vi "Get Conditional Column Data.vi"(4 "Condition Header Value":string, 6 "Condition Header":string, 8 "error in (no error)":errorcluster, 10 "Header":string, 11 "SLL Table in":refnum<class "SLL Table.lvclass">) -> (0 "error out":errorcluster, 2 "Data[]":string[](array[string]), 3 "SLL Table out":refnum<class "SLL Table.lvclass">)   [LabVIEW 2014, in "SLL Table.lvclass"]
uses:
  SLL Table.lvclass
  SLL String/SLL String.lvlib
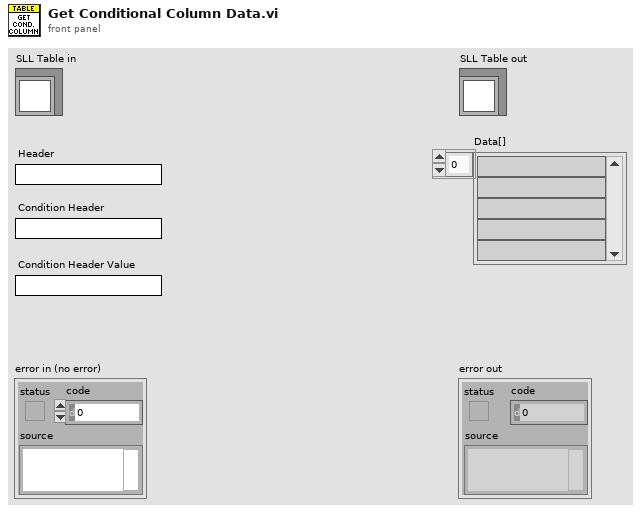
[diagram p1: front panel]
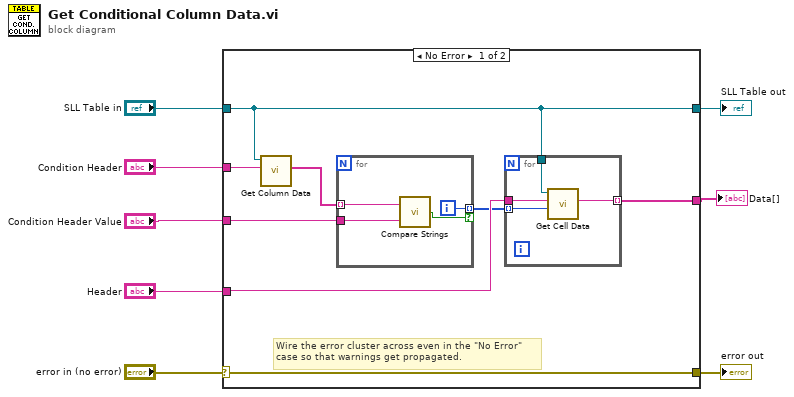
[diagram p0: block diagram]
diagram:
  n1 = case shown="No Error" "error in (no error)" {
    selector: "error in (no error)" -> [w16 w26]
    tunnel: [w16 w26] -> w7
    tunnel: [w14 w25] -> w5
    tunnel: "SLL Table in" -> [w14 w25]
    tunnel: "Header" -> [w13 _]
    tunnel: [w11 _] -> w3
    tunnel: "Condition Header" -> [w10 _]
    tunnel: "Condition Header Value" -> [w9 _]
    frame No Error {
      # "Wire the error cluster across even in the \"No Error\"\ncase so that warnings get propagated."
      n2 = call "Get Column Data.vi"("Header"=w10, "SLL Table in"=w14) -> ("Data[]"=w15:string[])  [unwired: 6 in, 3 out]
      n3 = for {
        tunnel: w15 -> [w24] mode=indexing
        tunnel: w9 -> [w23]
        tunnel: [w22] -> w12 mode=indexing if=w21
        i -> [w22]
        n4 = call "Compare Strings.vi"("y"=w23, "x"=w24) -> ("Equal?"=w21:bool)
      }
      n5 = for {
        tunnel: w14 -> [w20]
        tunnel: w13 -> [w19]
        tunnel: w12 -> [w18] mode=indexing
        tunnel: [w17] -> w11 mode=indexing
        n6 = call "Get Cell Data.vi"("Row Index"=w18, "Header"=w19, "SLL Table in"=w20) -> ("Cell Data"=w17:string)  [unwired: 5 in, 3 out]
      }
    }
    frame Error {
    }
  }
  "error out" <- w7
  "SLL Table out" <- w5
  "Data[]" <- w3
